vi "GetDataPackage_Variant.vi"(8 "error in (no error)":errorcluster, 11 "VISA Refnum in":refnum<visa-resource-name>) -> (0 "error out":errorcluster, 1 "Raw Data":string, 2 "Data":T1[](array[typedef]), 3 "VISA Refnum out":refnum<visa-resource-name>)   [LabVIEW 2020, in "OXYGEN_Datastream.lvlib"]
uses:
  OXYGEN_Datastream.lvlib
  TypeDefs/DataPoint_Variant.ctl
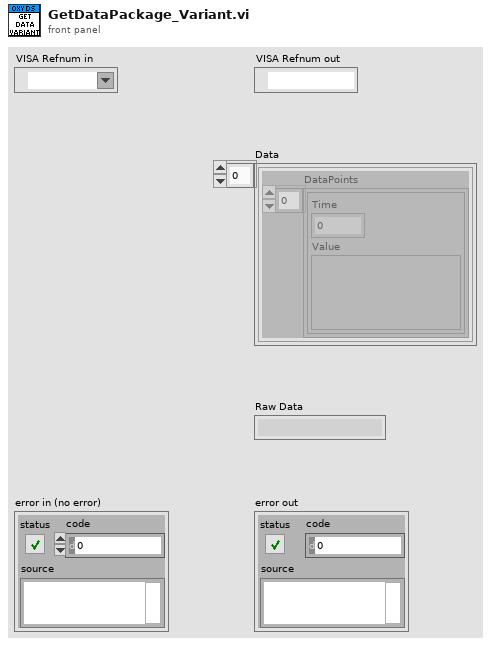
[diagram p1: front panel]
types:
  T1 = typedef "OXYGEN_Datastream.lvlib/DataPoint_Variant.ctl" = cluster{"DataPoints":cluster{"Time":dbl, "Value":variant}[]}
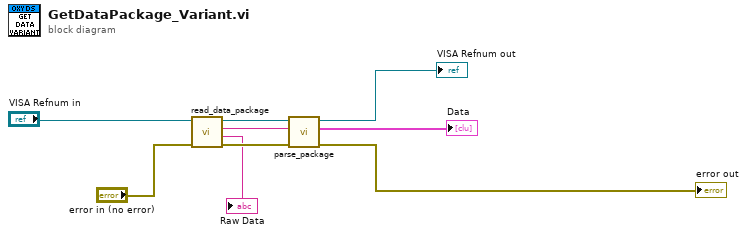
[diagram p0: block diagram]
diagram:
  n1 = call "read_data_package.vi"("error in (no error)"="error in (no error)", "OXY_SCPI Reseource In"="VISA Refnum in") -> ("error out"=w3:errorcluster, "Complete Raw data"=→"Raw Data":string, "Package without Header"=w5:string, "OXY_SCPI Reseource Out"=w4:refnum<visa-resource-name>)  [unwired: 6 in]
  n2 = call "parse_package.vi"("error in (no error)"=w3, "Raw Package without Header"=w5, "OXY_SCPI Reseource In"=w4) -> ("error out"=→"error out":errorcluster, "DataAllChannels"=→"Data":T1[], "OXY_SCPI Reseource Out"=→"VISA Refnum out":refnum<visa-resource-name>)  [unwired: 6 in]
